vi "Create Organization Price Comparison.vi"() -> ()   [LabVIEW 2010]
uses:
  <vilib>/Platform/browser.llb/Open URL in Default Browser (string).vi
panel:
  out "Boolean 2":bool
  out "Path 2":path
  out "Path":path
  out "String 2":string
  out "String":string
  out "concatenated string":string
  out "appended path":path
  out "Most Recent File Path":path
  out "name":string
  out "standard output 4":string
  out "error out 4":errorcluster
  out "standard error 4":string
  out "error out 3":errorcluster
  out "standard error 3":string
  out "standard output 3":string
  out "error out 2":errorcluster
  out "standard error 2":string
  out "standard output 2":string
  out "standard output":string
  out "error out":errorcluster
  out "standard error":string
  out "number 2":i32
  out "Boolean":bool
  out "number of replacements":i32
  in  "stop":bool
  out "number":i32
  out "Desired Extension":string
  out "Website":string
  out "E-mail":string
  out "Last Name":string
  out "First Name":string
  out "Logo Location":string
  out "Logo Name":string
  out "Organization Name":string
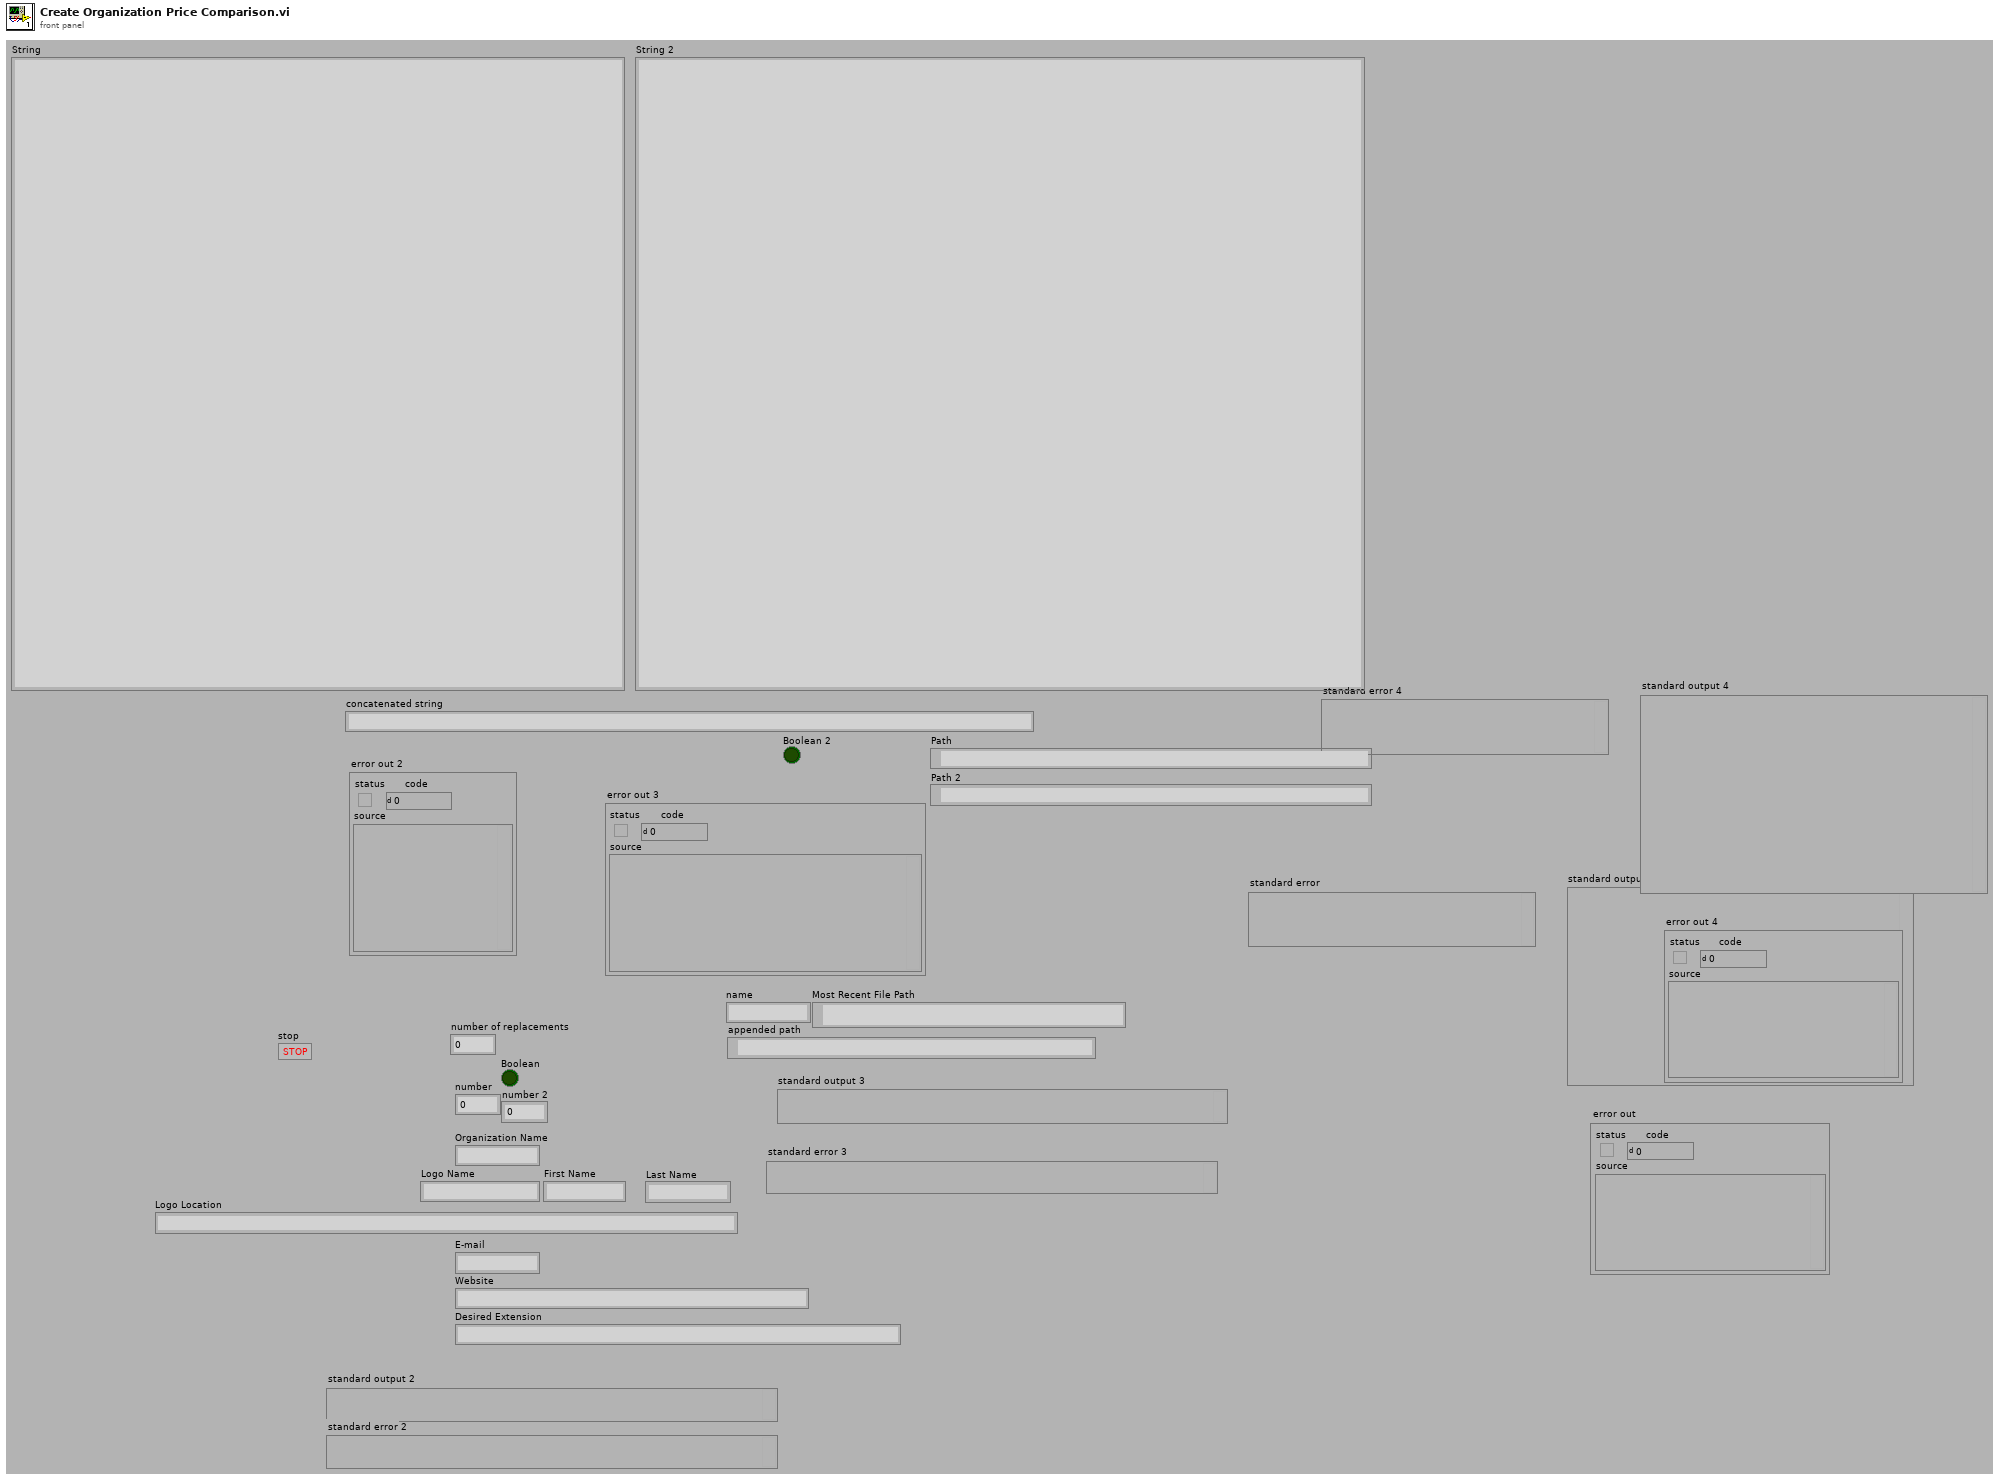
[diagram p1: front panel]
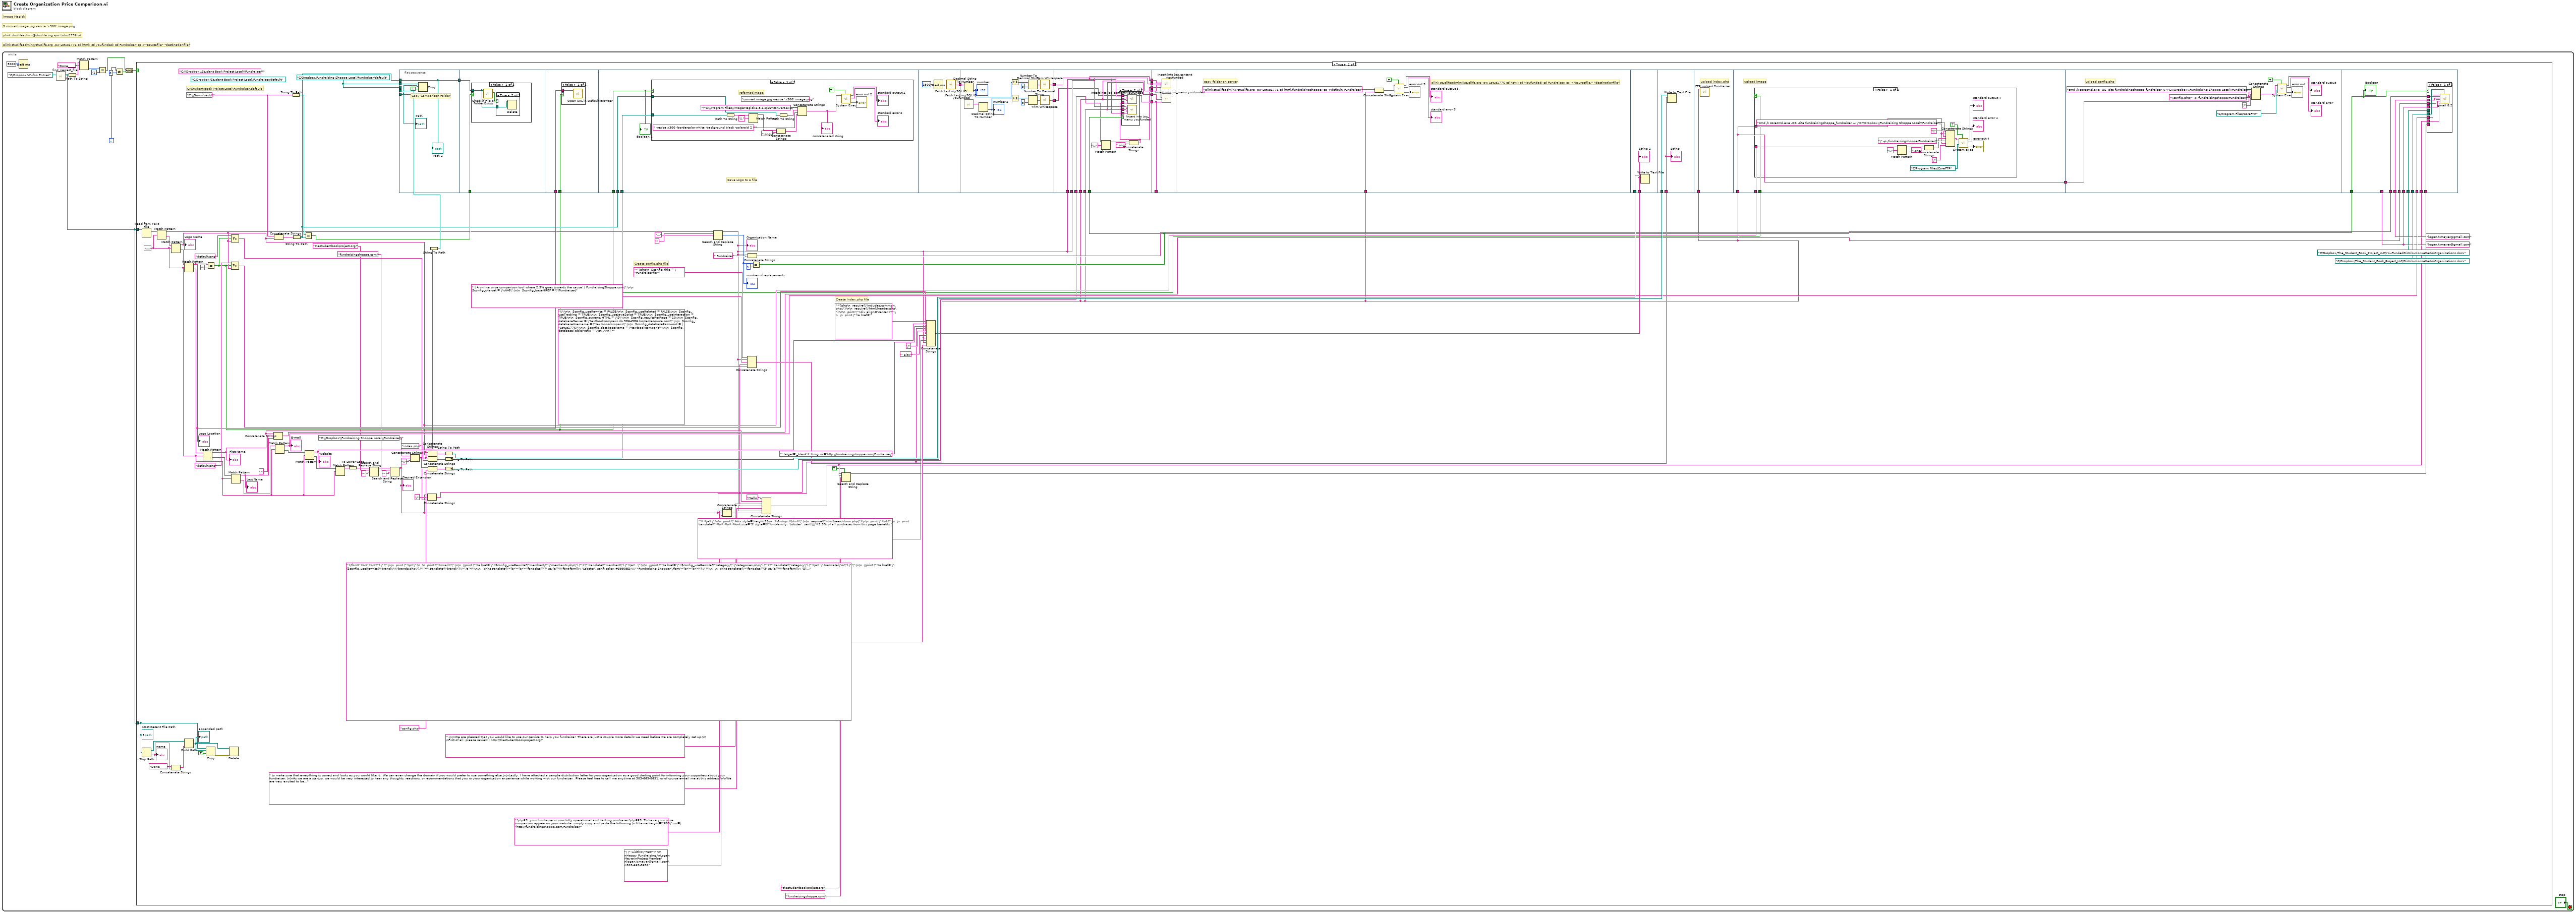
[diagram p0: block diagram]
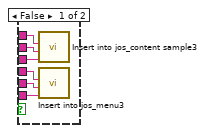
[diagram p7: hidden frame]
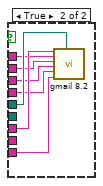
[diagram p9: hidden frame]
diagram:
  # "plink stuslifeadmin@stuslife.org -pw Lotus1776 cd html; cd youfunded; cd Fundraiser; cp -r *sourcefile* *destinationfile*"
  # "plink stuslifeadmin@stuslife.org -pw Lotus1776 cd"
  # "image Magick"
  # "$ convert image.jpg -resize 'x300' image.png"
  n1 = while {
    i -> [w12]
    stop <- "stop" stop-if-true
    n2 = Wait (ms)(milliseconds to wait=u32 5000) -> ()  [unwired: 1 out]
    n3 = call "find_newest_file.vi"("Directory Path to Start the Search"=path "C:/Dropbox/Wufoo Entries") -> ("Most Recent File Path"=w5:path)  [unwired: 9 in, 1 out]
    n4 = Path To String(path=w5) -> (string=w4:string)
    n5 = Match Pattern(string=w4, regular expression="Done_____") -> (offset past match=w7:i32)  [unwired: 1 in, 3 out]
    n6 = Equal?(x=w7, y=-1) -> (x = y?=w1:bool)
    n7 = Not Equal?(x=w12, y=0) -> (x != y?=w3:bool)
    n8 = And(x=w1, y=w3) -> (x .and. y?=w2:bool)
    n9 = case shown="True" w2 {
      tunnel: w5 -> [_ w119]
      tunnel: w5 -> [_ w17]
      frame False {
      }
      frame True {
        (unwired) "C:\\Dropbox\\Student Book Project Local\\Fundraiser\\" ("Source URL")
        (unwired) path "C:/Dropbox/Student Book Project Local/Fundraiser/default" ("source path")
        w49 = path "C:/Dropbox/Fundraising Shoppe Local/Fundraiser/default" ("source path")
        w69 = "C:\\Downloads\\" ("Source URL")
        w72 = "logan.t.meyer@gmail.com" ("CC (Carbon Copy Recipient - Optional)")
        w85 = "::::" ("search string/char (-)")
        # "C:\\Student Book Project Local\\Fundraiser\\default"
        # "Create Index.php file"
        # "Create config.php file"
        n10 = Read from Text File(file (use dialog)=w119) -> (text=w118:string)  [unwired: 3 in, 3 out]
        n11 = Strip Path(path=w17) -> (stripped path=w22:path, name=w23:string)
        "name" <- w23
        n12 = Match Pattern(string=w118, regular expression=w85) -> (before substring=w54:string, after substring=w117:string)  [unwired: 1 in, 2 out]
        n13 = Match Pattern(string=w117, regular expression=w85) -> (before substring=w16:string, after substring=w116:string)  [unwired: 1 in, 2 out]
        "Logo Name" <- w16
        n14 = Concatenate Strings("Done_____" ("regular expression"), w23) -> (w21:string)
        n15 = Match Pattern(string=w116, regular expression=w85) -> (before substring=w70:string, after substring=w115:string)  [unwired: 1 in, 2 out]
        "Logo Location" <- w70
        n16 = Build Path(base path=w22, name or relative path=w21) -> (appended path=w20:path)
        "appended path" <- w20
        n17 = Match Pattern(string=w115, regular expression=w85) -> (before substring=w94:string, after substring=w114:string)  [unwired: 1 in, 2 out]
        "First Name" <- w94
        n18 = Copy(9:TRUE ("overwrite (F)"), 10:w20, 11:w17) -> (0:w18:errorcluster)  [unwired: 2 in, 2 out]
        n19 = Equal?(x=w70, y="") -> (x = y?=w14:bool)
        n20 = Delete(path (use dialog)=w17, error in=w18) -> ()  [unwired: 3 in, 3 out]
        n21 = Select(t="default.png", s=w14, f=w16) -> (s? t:f=w60:string)
        n22 = Select(t="default.png", s=w14, f=w16) -> (s? t:f=w64:string)
        n23 = Match Pattern(string=w114, regular expression=w85) -> (before substring=w92:string, after substring=w113:string)  [unwired: 1 in, 2 out]
        "Last Name" <- w92
        n24 = Concatenate Strings(w94, " " ("string"), w92) -> (w73:string)
        n25 = Concatenate Strings(w69, w16) -> (w88:string)
        n26 = Match Pattern(string=w113, regular expression=w85) -> (before substring=w76:string, after substring=w112:string)  [unwired: 1 in, 2 out]
        "E-mail" <- w76
        n27 = String To Path(string=w69) -> (path=w67:path)
        n28 = String To Path(string=w88) -> (path=w68:path)
        n29 = Equal?(x=w67, y=w68) -> (x = y?=w66:bool)
        n30 = Match Pattern(string=w112, regular expression=w85) -> (before substring=w104:string, after substring=w86:string)  [unwired: 1 in, 2 out]
        "Website" <- w104
        n31 = Match Pattern(string=w86, regular expression=w85) -> (before substring=w83:string)  [unwired: 1 in, 3 out]
        n32 = To Lower Case(string=w83) -> (all lower case string=w29:string)
        n33 = Search and Replace String(input string=w29, search string="thestudentbookproject.org/", replace string="" ("replace string (\"\")")) -> (result string=w28:string)  [unwired: 5 in, 3 out]
        n34 = Search and Replace String(input string=w28, search string="fundraisingshoppe.com/", replace string="" ("replace string (\"\")")) -> (result string=w15:string)  [unwired: 5 in, 3 out]
        "Desired Extension" <- w15
        n35 = flat-sequence {
          tunnel: w68 -> [w123]
          tunnel: [w123] -> w82
          tunnel: w49 -> [_]
          tunnel: w62 -> [_]
          tunnel: w49 -> [w121]
          tunnel: w62 -> [w120]
          tunnel: w82 -> [w125]
          tunnel: w66 -> [w124]
          tunnel: w70 -> [w130]
          tunnel: w14 -> [w129]
          tunnel: w87 -> [w134]
          tunnel: w68 -> [w133]
          tunnel: w14 -> [w132]
          tunnel: [w150] -> w36
          tunnel: [w154] -> w39
          tunnel: [w153] -> w37
          tunnel: w36 -> [w152]
          tunnel: w53 -> [w172]
          tunnel: w59 -> [w165]
          tunnel: w15 -> [w171]
          tunnel: w53 -> [w174]
          tunnel: w15 -> [w173]
          tunnel: w51 -> [w175]
          tunnel: [w174] -> w44
          tunnel: [w173] -> w43
          tunnel: [w172] -> w42
          tunnel: [w171] -> w41
          tunnel: [w164] -> w40
          tunnel: w39 -> [w170]
          tunnel: [w169] -> w38
          tunnel: w37 -> [w169]
          tunnel: w44 -> [w193]
          tunnel: w43 -> [w192]
          tunnel: w42 -> [w191]
          tunnel: w41 -> [w190]
          tunnel: w40 -> [w189]
          tunnel: [w188] -> _
          tunnel: w38 -> [w188]
          tunnel: w15 -> [w195]
          tunnel: w81 -> [w202]
          tunnel: w80 -> [w201]
          tunnel: w79 -> [w204]
          tunnel: w78 -> [w203]
          tunnel: w15 -> [w205]
          tunnel: [w207] -> w25
          tunnel: w16 -> [w208]
          tunnel: w15 -> [w207]
          tunnel: w14 -> [w206]
          tunnel: w25 -> [w225]
          tunnel: path "C:/Dropbox/The_Student_Book_Project_LLC/DistributionLetterforOrganizations.docx" ("Attachment - Optional") -> [w244]
          tunnel: w76 -> [w238]
          tunnel: w75 -> [w243]
          tunnel: "logan.t.meyer@gmail.com" ("Sender's Email Address (eg: jsmith77@gmail.com)") -> [w241]
          tunnel: w72 -> [_]
          tunnel: w48 -> [w242]
          tunnel: w73 -> [w240]
          tunnel: w72 -> [w239]
          tunnel: path "C:/Dropbox/The_Student_Book_Project_LLC/YouFundedDistributionLetterforOrganizations.docx" ("Attachment - Optional") -> [w237]
          tunnel: w51 -> [w236]
          tunnel: w45 -> [w235]
          frame #0 {
            # "Copy Comparison Folder"
            n36 = Copy(9:TRUE ("overwrite (F)"), 10:w120, 11:w121) -> ()  [unwired: 2 in, 3 out]
            "Path" <- w120
            "Path 2" <- w123
          }
          frame #1 {
            n37 = case shown="False" w124 {
              tunnel: w125 -> [w126 _]
              frame False {
                n38 = call <vilib>:"Check if File or Folder Exists.vi"("path"=w126) -> ("file or folder exists?"=w127:bool)  [unwired: 8 in, 2 out]
                n39 = case shown="True" w127 {
                  tunnel: w126 -> [_ w128]
                  frame False {
                  }
                  frame True {
                    n40 = Delete(path (use dialog)=w128) -> ()  [unwired: 4 in, 3 out]
                  }
                }
              }
              frame True {
              }
            }
          }
          frame #2 {
            n41 = case shown="False" w129 {
              tunnel: w130 -> [w131 _]
              frame False {
                n42 = call-poly <vilib>:"Open URL in Default Browser.vi"("URL"=w131) -> ()  [unwired: 5 in, 2 out]
              }
              frame True {
              }
            }
          }
          frame #3 {
            # "Save Logo to a file"
            n43 = case shown="False" w132 {
              tunnel: w134 -> [w145 _]
              tunnel: w133 -> [w146 _]
              frame False {
                (unwired) "convert image.jpg -resize 'x300' image.png" ("command line")
                # "reformat image"
                n44 = Path To String(path=w145) -> (string=w141:string)
                n45 = Match Pattern(string=w141, regular expression="\\.") -> (before substring=w139:string)  [unwired: 1 in, 3 out]
                n46 = Concatenate Strings(w139, ".png\"" ("string")) -> (w135:string)
                n47 = Path To String(path=w146) -> (string=w144:string)
                n48 = Concatenate Strings("\"C:\\Program Files\\ImageMagick-6.8.1-Q16\\convert.exe\" " ("string"), w144, " -resize x300 -bordercolor white -background black -polaroid 2 \"" ("string"), w135) -> (w140:string)
                "concatenated string" <- w140
                n49 = call <vilib>:"System Exec.vi"("wait until completion? (T)"=TRUE, "command line"=w140) -> ("error out"=→"error out 2":errorcluster, "standard error"=→"standard error 2":string, "standard output"=→"standard output 2":string)  [unwired: 6 in, 1 out]
              }
              frame True {
              }
            }
            "Boolean 2" <- w132
          }
          frame #4 {
            n50 = Wait (ms)(milliseconds to wait=u32 1500) -> ()  [unwired: 1 out]
            n51 = call "Fetch Last mySQL ID.vi"() -> ("Last ID"=w150:string)  [unwired: 1 in]
          }
          frame #5 {
            n52 = Decimal String To Number(string=w152) -> (number=w160:i32)  [unwired: 2 in, 1 out]
            "number" <- w160
            n53 = call "Fetch Last mySQL ID youfunded.vi"() -> ("Last ID"=w159:string)  [unwired: 1 in]
            n54 = Decimal String To Number(string=w159) -> (number=w155:i32)  [unwired: 2 in, 1 out]
            "number 2" <- w155
            n55 = Increment(x=w160) -> (x+1=w161:i32)
            n56 = Increment(x=w155) -> (x+1=w156:i32)
            n57 = Number To Decimal String(number=w161, width (-)=i16 5) -> (decimal integer string=w162:string)
            n58 = Number To Decimal String(number=w156, width (-)=i16 5) -> (decimal integer string=w158:string)
            n59 = call <vilib>:"Trim Whitespace.vi"("string"=w162) -> ("trimmed string"=w154:string)  [unwired: 1 in]
            n60 = call <vilib>:"Trim Whitespace.vi"("string"=w158) -> ("trimmed string"=w153:string)  [unwired: 1 in]
          }
          frame #6 {
            n61 = Match Pattern(string=w165, regular expression="\\.") -> (before substring=w166:string)  [unwired: 1 in, 3 out]
            n62 = Concatenate Strings(w166, ".png" ("string")) -> (w164:string)
            n63 = case shown="True" w175 {
              tunnel: w174 -> [w181 w182]
              tunnel: w173 -> [w180 w183]
              tunnel: w170 -> [w179 w184]
              tunnel: w172 -> [w178 w186]
              tunnel: w171 -> [w177 w185]
              tunnel: w164 -> [w176 w187]
              frame False {
                n64 = call "Insert into jos_content sample3.vi"("Logo Name"=w176, "alias"=w177, "title"=w178) -> ()  [unwired: 2 in]
                n65 = call "Insert into jos_menu3.vi"("id of content article"=w179, "alias"=w180, "title"=w181) -> ()  [unwired: 2 in]
              }
              frame True {
                n66 = call "Insert into jos_content youfunded.vi"("Logo Name"=w187, "alias"=w185, "title"=w186) -> ()  [unwired: 2 in]
                n67 = call "Insert into jos_menu youfunded.vi"("id of content article"=w184, "alias"=w183, "title"=w182) -> ()  [unwired: 2 in]
              }
            }
          }
          frame #7 {
            n68 = call "Insert into jos_content youfunded.vi"("Logo Name"=w189, "alias"=w190, "title"=w191) -> ()  [unwired: 2 in]
            n69 = call "Insert into jos_menu youfunded.vi"("id of content article"=w188, "alias"=w192, "title"=w193) -> ()  [unwired: 2 in]
          }
          frame #8 {
            # "copy folder on server"
            # "plink stuslifeadmin@stuslife.org -pw Lotus1776 cd html; cd youfunded; cd Fundraiser; cp -r *sourcefile/* *destinationfile*"
            n70 = Concatenate Strings("plink stuslifeadmin@stuslife.org -pw Lotus1776 cd html/fundraisingshoppe; cp -r default/ Fundraiser/" ("string"), w195) -> (w196:string)
            n71 = call <vilib>:"System Exec.vi"("wait until completion? (T)"=TRUE, "command line"=w196) -> ("error out"=→"error out 3":errorcluster, "standard error"=→"standard error 3":string, "standard output"=→"standard output 3":string)  [unwired: 6 in, 1 out]
          }
          frame #9 {
            n72 = Write to Text File(file (use dialog)=w202, text=w201) -> ()  [unwired: 2 in, 3 out]
            "String 2" <- w201
          }
          frame #10 {
            n73 = Write to Text File(file (use dialog)=w204, text=w203) -> ()  [unwired: 2 in, 3 out]
            "String" <- w203
          }
          frame #11 {
            # "upload index.php"
            n74 = call "FTP upload Fundraiser.vi"("extension"=w205) -> ()  [unwired: 11 in]
          }
          frame #12 {
            # "upload image"
            n75 = case shown="False" w206 {
              tunnel: w208 -> [w210 _]
              tunnel: w207 -> [w212 _]
              frame False {
                n76 = Match Pattern(string=w210, regular expression="\\.") -> (before substring=w209:string)  [unwired: 1 in, 3 out]
                n77 = Concatenate Strings(w209, ".png" ("string")) -> (w213:string)
                n78 = Concatenate Strings("cmd /k corecmd.exe -OS -site fundraisingshoppe_fundraiser -u \"C:\\Dropbox\\Fundraising Shoppe Local\\Fundraiser\\" ("string"), w212, "\\" ("string"), w213, "\" -p /fundraisingshoppe/Fundraiser/" ("string"), w212, "/" ("string")) -> (w218:string)
                n79 = call <vilib>:"System Exec.vi"("wait until completion? (T)"=TRUE, "working directory"=path "C:/Program Files/CoreFTP", "command line"=w218) -> ("error out"=→"error out 4":errorcluster, "standard error"=→"standard error 4":string, "standard output"=→"standard output 4":string)  [unwired: 5 in, 1 out]
              }
              frame True {
              }
            }
          }
          frame #13 {
            # "upload config.php"
            n80 = Concatenate Strings("cmd /k corecmd.exe -OS -site fundraisingshoppe_fundraiser -u \"C:\\Dropbox\\Fundraising Shoppe Local\\Fundraiser\\" ("string"), w225, "\\config.php\" -p /fundraisingshoppe/Fundraiser/" ("string"), w225, "/" ("string")) -> (w227:string)
            n81 = call <vilib>:"System Exec.vi"("wait until completion? (T)"=TRUE, "working directory"=path "C:/Program Files/CoreFTP", "command line"=w227) -> ("error out"=→"error out":errorcluster, "standard error"=→"standard error":string, "standard output"=→"standard output":string)  [unwired: 5 in, 1 out]
          }
          frame #14 {
            n82 = case shown="False" w236 {
              tunnel: w244 -> [w251 _]
              tunnel: w243 -> [w250 w255]
              tunnel: w242 -> [w249 _]
              tunnel: w241 -> [w248 w254]
              tunnel: w240 -> [w247 w253]
              tunnel: w239 -> [w246 w252]
              tunnel: w238 -> [w245 w256]
              tunnel: w237 -> [_ w258]
              tunnel: w235 -> [_ w257]
              frame False {
                n83 = call "gmail 8.2.vi"("Recipient's Email Address Address"=w245, "Subject"=w250, "Sender's Email Address (eg: jsmith77@gmail.com)"=w248, "Recipient's Name"=w247, "CC (Carbon Copy Recipient - Optional)"=w246, "Body"=w249, "Attachment - Optional"=w251) -> ()  [unwired: 13 in]
              }
              frame True {
                n84 = call "gmail 8.2.vi"("Recipient's Email Address Address"=w256, "Subject"=w255, "Sender's Email Address (eg: jsmith77@gmail.com)"=w254, "Recipient's Name"=w253, "CC (Carbon Copy Recipient - Optional)"=w252, "Body"=w257, "Attachment - Optional"=w258) -> ()  [unwired: 13 in]
              }
            }
            "Boolean" <- w236
          }
        }
        n85 = Concatenate Strings("C:\\Dropbox\\Fundraising Shoppe Local\\Fundraiser\\" ("Source URL"), w15, "\\" ("string")) -> (w90:string)
        n86 = Concatenate Strings(w15, "/" ("string"), w60) -> (w59:string)
        n87 = Concatenate Strings(w90, w16) -> (w89:string)
        n88 = Concatenate Strings(w90, "index.php" ("string")) -> (w99:string)
        n89 = Concatenate Strings(w90, "config.php" ("string")) -> (w106:string)
        n90 = String To Path(string=w90) -> (path=w62:path)
        n91 = String To Path(string=w89) -> (path=w87:path)
        n92 = String To Path(string=w99) -> (path=w81:path)
        n93 = String To Path(string=w106) -> (path=w79:path)
        n94 = Search and Replace String(input string=w54, search string="---", replace string="" ("replace string (\"\")")) -> (result string=w53:string, number of replacements=w56:i32)  [unwired: 5 in, 2 out]
        "Organization Name" <- w53
        "number of replacements" <- w56
        n95 = Concatenate Strings("!\n\nPS, your fundraiser is now fully operational and tracking purchases!\n\nPPS, To have your price comparison appear on your website, simply copy and paste the following:\n<iframe height=\"600\" src=\"http://fundraisingshoppe.com/Fundraiser/" ("string"), w15, "/ \" width=\"760\"> \n\nHappy Fundraising,\nLogan Meyer\nProject Member\nlogan.t.meyer@gmail.com\n303-669-8691" ("string")) -> (w33:string)
        n96 = Concatenate Strings("<?php\n  $config_title = \"Fundraiser for ", w53, " | A online price comparison tool where 2.5% goes towards the cause! | FundraisingShoppe.com\";\n\n  $config_charset = \"utf-8\";\n\n  $config_baseHREF = \"/Fundraiser/" ("string"), w15, "/\";\n\n  $config_useRewrite = FALSE;\n\n  $config_useRelated = FALSE;\n\n  $config_useTracking = TRUE;\n\n  $config_useJavaScript = TRUE;\n\n  $config_useInteraction = TRUE;\n\n  $config_currencyHTML = \"$\";\n\n  $config_resultsPerPage = 10;\n\n  $config_databaseServer = \"textbookcomparis.db.5864586.hostedresource.com\";\n\n  $config_databaseUsername = \"textbookcomparis\";\n\n  $config_databasePassword = \"Lotus1776\";\n\n  $config_databaseName = \"textbookcomparis\";\n\n  $config_databaseTablePrefix = \"pt_\";\n?>" ("string")) -> (w78:string)
        n97 = Concatenate Strings(w53, " Fundraiser" ("string")) -> (w75:string)
        n98 = Equal?(x=w56, y=1) -> (x = y?=w51:bool)
        n99 = Concatenate Strings("Hello ", w94, ",\n\nWe are pleased that you would like to use our service to help you fundraise!  There are just a couple more details we need before we are completely set up.\n\nFirst of all, please review : http://thestudentbookproject.org/" ("string"), w15, " to make sure that everything is correct and looks as you would like it.  We can even change the domain if you would prefer to use something else.\n\nLastly, I have attached a sample distribution letter for your organization as a good starting point for informing your supporters about your fundraiser. \n\nAs we are a startup, we would be very interested to hear any thoughts, reactions, or recommendations that you or your organization experience while working with our fundraiser.  Please feel free to call me anytime at 303-669-8691, or of course e-mail me at this address.\n\nWe are very excited to be working with " ("string"), w53, w33) -> (w48:string)
        n100 = Search and Replace String(replace all?=TRUE ("replace all? (F)"), input string=w48, search string="thestudentbookproject.org", replace string="fundraisingshoppe.com" ("replace string (\"\")")) -> (result string=w45:string)  [unwired: 4 in, 3 out]
        n101 = Concatenate Strings("<?php\n  require(\"includes/common.php\");\n\n  require(\"html/header.php\");\n\n  print \"<div align='center'>\";\n  \n  print \"<a href='", w104, "' target='_blank'><img src='http://fundraisingshoppe.com/Fundraiser/" ("string"), w15, "/" ("string"), w64, "' alt='" ("string"), w53, "'></a>\";\n\n  print \"<div style='height:20px;'>&nbsp;</div>\";\n\n  require(\"html/searchform.php\");\n\n  print \"<p>\";\n  \n  print translate(\"<br><br><font size='5' style=\\\"font-family: 'Lobster', serif;\\\">2.5% of all purchases from this page benefits " ("string"), w53, "</font><br><br>\").\" \";\n\n  print \"<p>\";\n  \n  print \"<small>\";\n\n  //print \"<a href='\".($config_useRewrite?\"merchant/\":\"merchants.php\").\"'>\".translate(\"merchant\").\"</a>, \";\n\n  //print \"<a href='\".($config_useRewrite?\"category/\":\"categories.php\").\"'>\".translate(\"category\").\"</a> \".translate(\"or\").\" \";\n\n  //print \"<a href='\".($config_useRewrite?\"brand/\":\"brands.php\").\"'>\".translate(\"brand\").\"</a>\";\n\n   print translate(\"<br><br><font size='7' style=\\\"font-family: 'Lobster', serif; color: #3990BD;\\\">Fundraising Shoppe</font><br><br>\").\" \";\n  \n  print translate(\"<font size='3' style=\\\"font-family: 'Didact Gothic', serif;\\\">Compare on any and all products!</font>\").\" \";\n  \n  print translate(\"<br><font size='2' style=\\\"font-family: 'Didact Gothic', serif;\\\">Can't find your fundraiser?  <a href='http://thestudentbookproject.org/fundraise.html' target='_blank'>Start one</a> today at <a href='http://fundraisingshoppe.com/fundraise.html' target='_blank'>fundraisingshoppe.com</a>!</font>\").\" \";\n  \n  print \"</small>\";\n\n  print \"</p>\";\n\n  print \"</div>\";\n\n  print javascript_focus(\"search.q\");\n\n  $sql = \"SELECT * FROM `\".$config_databaseTablePrefix.\"featured` ORDER BY sequence\";\n\n  if (database_querySelect($sql,$rows))\n  {\n    $sqlNames = array();\n\n    $sqlCase = \"CASE normalised_name\";\n\n    foreach($rows as $featured)\n    {\n      $featured[\"name\"] = tapestry_normalise($featured[\"name\"]);\n\n      $sqlNames[] = \"'\".$featured[\"name\"].\"'\";\n\n      $sqlCase .= \" WHEN '\".database_safe($featured[\"name\"]).\"' THEN \".$featured[\"sequence\"];\n    }\n\n    $sqlCase .= \" END AS sequence\";\n\n    $sqlIn = implode(\",\",$sqlNames);\n\n    $sql = \"SELECT * , MIN( price ) AS minPrice, MAX( price ) AS maxPrice, COUNT( id ) AS numMerchants, \".$sqlCase.\" FROM `\".$config_databaseTablePrefix.\"products` WHERE normalised_name IN (\".$sqlIn.\") GROUP BY normalised_name ORDER BY sequence\";\n\n    database_querySelect($sql,$rows);\n\n    $featured[\"products\"] = $rows;\n\n    foreach($featured[\"products\"] as $k => $product)\n    {\n      $featured[\"products\"][$k][\"productHREF\"] = tapestry_productHREF($product);\n\n      $featured[\"products\"][$k][\"reviewHREF\"] = tapestry_reviewHREF($product);\n    }\n  }\n\n  if (isset($featured)) require(\"html/featured.php\");\n\n  require(\"html/footer.php\");\n?>" ("string")) -> (w80:string)
        "Most Recent File Path" <- w17
      }
    }
  }
